vi "lvstyx_write_path_int.vi"(7 "Log? (T)":bool=TRUE, 8 "error in (no error)":errorcluster, 9 "int64":i64, 10 "path":string, 11 "client ptr":u32) -> (0 "error out":errorcluster, 3 "dup client ptr":u32)   [LabVIEW 2010, in "lib1299.lvlib"]
uses:
  lib1299.lvlib
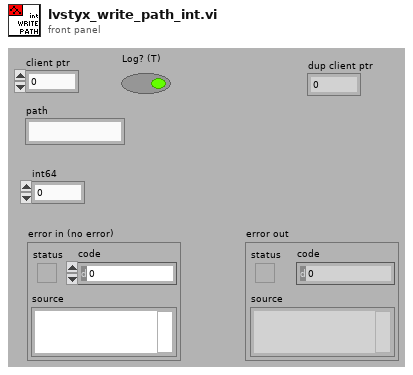
[diagram p1: front panel]
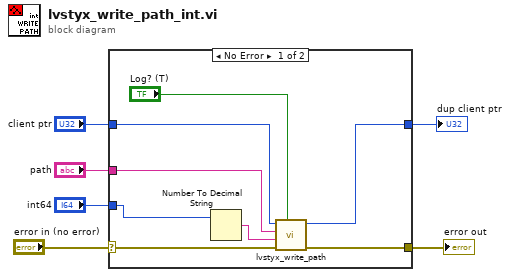
[diagram p0: block diagram]
diagram:
  n1 = case shown="No Error" "error in (no error)" {
    selector: "error in (no error)" -> [w13 w16]
    tunnel: [w14 w16] -> w6
    tunnel: "int64" -> [w11 _]
    tunnel: "path" -> [w10 _]
    tunnel: "client ptr" -> [w9 w15]
    tunnel: [w8 w15] -> w1
    frame No Error {
      n2 = Number To Decimal String(number=w11) -> (decimal integer string=w12:string)  [unwired: 1 in]
      n3 = call "lvstyx_write_path.vi"("Log? (T)"="Log? (T)", "error in (no error)"=w13, "buf"=w12, "path"=w10, "client ptr"=w9) -> ("error out"=w14:errorcluster, "dup client ptr"=w8:u32)  [unwired: 4 in, 1 out]
    }
    frame Error {
    }
  }
  "error out" <- w6
  "dup client ptr" <- w1
